vi "Write OUR.vi"(8 "error in (no error)":errorcluster, 10 "OUR":dbl, 11 "OUR_Monitor in":refnum<class "OUR_Monitor.lvclass">) -> (0 "error out":errorcluster, 3 "OUR_Monitor out":refnum<class "OUR_Monitor.lvclass">)   [LabVIEW 2021, in "MBPOnOff_Controller.lvlib" / "OUR_Monitor.lvclass"]
uses:
  OUR_Monitor.lvclass
  OUR_Monitor.lvclass/OUR_Monitor.ctl
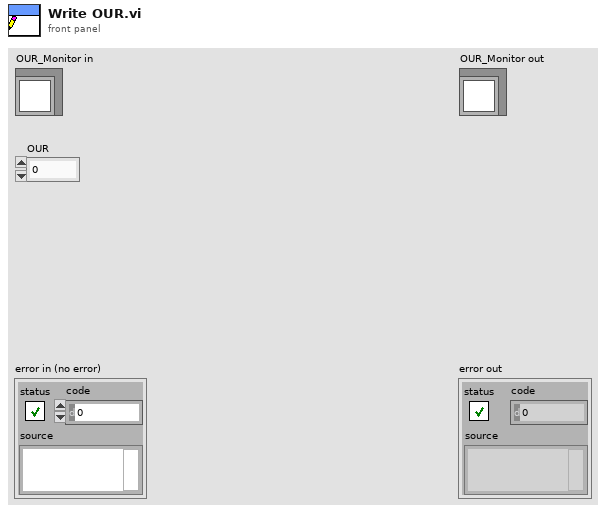
[diagram p1: front panel]
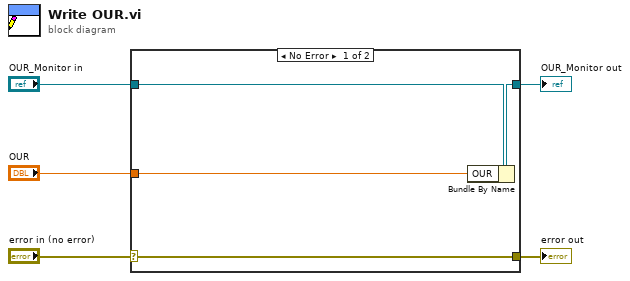
[diagram p0: block diagram]
diagram:
  n1 = case shown="No Error" "error in (no error)" {
    selector: "error in (no error)" -> [w9 w10]
    tunnel: [w9 w10] -> w4
    tunnel: [w7 w11] -> w2
    tunnel: "OUR_Monitor in" -> [w8 w11]
    tunnel: "OUR" -> [w6 _]
    frame No Error {
      n2 = Bundle By Name(cluster=w8, "OUR"=w6) -> (w7:refnum<class "OUR_Monitor.lvclass">)
    }
    frame Error {
    }
  }
  "error out" <- w4
  "OUR_Monitor out" <- w2
